vi "External Register Updated.vi"(4 "Register Value(s)":u16[](array[numeric]), 6 "String Value":string, 8 "error in (no error)":errorcluster, 9 "Value":dbl, 10 "Label":string, 11 "MB Slave in":refnum<class "Battery Pack.lvclass">) -> (0 "error out":errorcluster, 2 "Debug Cluster":cluster{string, string, "Value":dbl}, 3 "MB Slave out":refnum<class "Battery Pack.lvclass">)   [LabVIEW 2021, in "Battery Pack.lvclass"]
uses:
  Battery Pack.lvclass
  C:/Program Files (x86)/National Instruments/LabVIEW 2021/user.lib/S2 Labs/Module Framework/Modules/Base/Module.lvclass
  C:/Program Files (x86)/National Instruments/LabVIEW 2021/user.lib/S2 Labs/Module Framework/Modules/Modbus/Modbus Slave Base/Modbus Slave Base.lvclass
  <userlib>/S2 Labs/Queued State Machine/TypeDefs/Queue Message.ctl
  <userlib>/S2 Labs/Queued State Machine/TypeDefs/States.ctl
  <userlib>/S2 Labs/Module Framework/Modules/Base/Module.lvclass/Module.ctl
  <userlib>/S2 Labs/Queued State Machine/QSM.lvclass/QSM.ctl
  <userlib>/S2 Labs/Module Framework/Modules/Modbus/Modbus Slave Base/Modbus Slave Base.lvclass/Modbus Slave Base.ctl
  3c32b7f4-6e0b-45a0-8bc8-92411707fda7.vi
  a5158770-3295-4c9c-bae0-3194b8534535.vi
  f352f066-f63e-40b9-9452-5cd8e12a8467.vi
  5f4802e9-4a10-4382-9869-df42cea41124.vi
  <userlib>/S2 Labs/Module Framework/Modules/Base/Read Name.vi
  <userlib>/S2 Labs/Module Framework/Modules/Modbus/Modbus Slave Base/Read MB Ref.vi
  b984352d-4769-4dd1-9690-e9a5a354050f.vi
  0fd58ad7-8179-4fbb-beb2-807b76c45ab5.vi
  fadbf1c2-6df0-41ab-86c2-22b80328d9ad.vi
  a5158770-3295-4c9c-bae0-3194b8534535.vi/a5442550-30ab-4f7c-a4e8-4e040bcf3d57.vi
  <userlib>/S2 Labs/Module Framework/Modules/Base/Read Queue.vi
  a5158770-3295-4c9c-bae0-3194b8534535.vi/77abbf80-a0d7-431e-91bd-d2268efe8bf3.vi
  a5158770-3295-4c9c-bae0-3194b8534535.vi/7a27d807-84e4-485a-8ba6-289735576614.vi
  5f4802e9-4a10-4382-9869-df42cea41124.vi/a5442550-30ab-4f7c-a4e8-4e040bcf3d57.vi
  5f4802e9-4a10-4382-9869-df42cea41124.vi/77abbf80-a0d7-431e-91bd-d2268efe8bf3.vi
  5f4802e9-4a10-4382-9869-df42cea41124.vi/7a27d807-84e4-485a-8ba6-289735576614.vi
  0fd58ad7-8179-4fbb-beb2-807b76c45ab5.vi/a5442550-30ab-4f7c-a4e8-4e040bcf3d57.vi
  0fd58ad7-8179-4fbb-beb2-807b76c45ab5.vi/77abbf80-a0d7-431e-91bd-d2268efe8bf3.vi
  0fd58ad7-8179-4fbb-beb2-807b76c45ab5.vi/7a27d807-84e4-485a-8ba6-289735576614.vi
  fadbf1c2-6df0-41ab-86c2-22b80328d9ad.vi/a5442550-30ab-4f7c-a4e8-4e040bcf3d57.vi
  fadbf1c2-6df0-41ab-86c2-22b80328d9ad.vi/77abbf80-a0d7-431e-91bd-d2268efe8bf3.vi
  fadbf1c2-6df0-41ab-86c2-22b80328d9ad.vi/7a27d807-84e4-485a-8ba6-289735576614.vi
  <userlib>/S2 Labs/Queued State Machine/Enqueue Element.vi
  <userlib>/S2 Labs/Module Framework/Modules/Base/Get Module Queues Map.vi
  <userlib>/S2 Labs/Queued State Machine/Callback Notifier/Obtain Callback Notifier.vi
  <userlib>/S2 Labs/Queued State Machine/Callback Notifier/Release Reply Notifier.vi
  <vilib>/JDP Science/JSONtext/Variant to JSON Text.vi
  <userlib>/S2 Labs/Alarms and Events Toolkit/Alarms/Set User Event.vi
  <userlib>/S2 Labs/Queued State Machine/QSM.lvclass
  <userlib>/S2 Labs/Queued State Machine/Callback Notifier/Callback Notifier.lvclass
  <vilib>/JDP Science/JSONtext/LVClass Serializer/JSONtext LVClass Serializer.lvclass
  <userlib>/S2 Labs/Modbus Toolkit/Slave/S2L Modbus Slave.lvclass
  MB Slave Simulator Base/MB Slave Simulator Base.lvclass
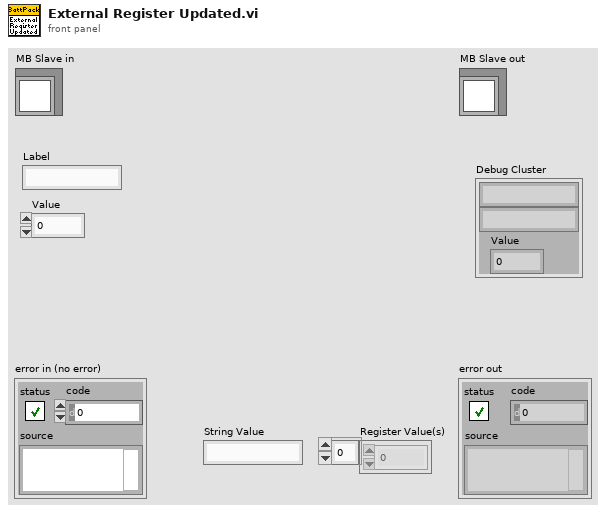
[diagram p1: front panel]
types:
  T1 = typedef "QSM.lvclass/Queue Message.ctl" = cluster{"State":T2, "Command":string, "Parameter":variant}
  T2 = typedef "QSM.lvclass/States.ctl" = enum16{"Waiting", "Init", "ExecCMD", "Read Config", "Write Config", "Launch", "Connect", "Recovery", "Clean Up", "Exit"}
  T3 = cluster{"Debug Message":string, string, "Value":dbl}
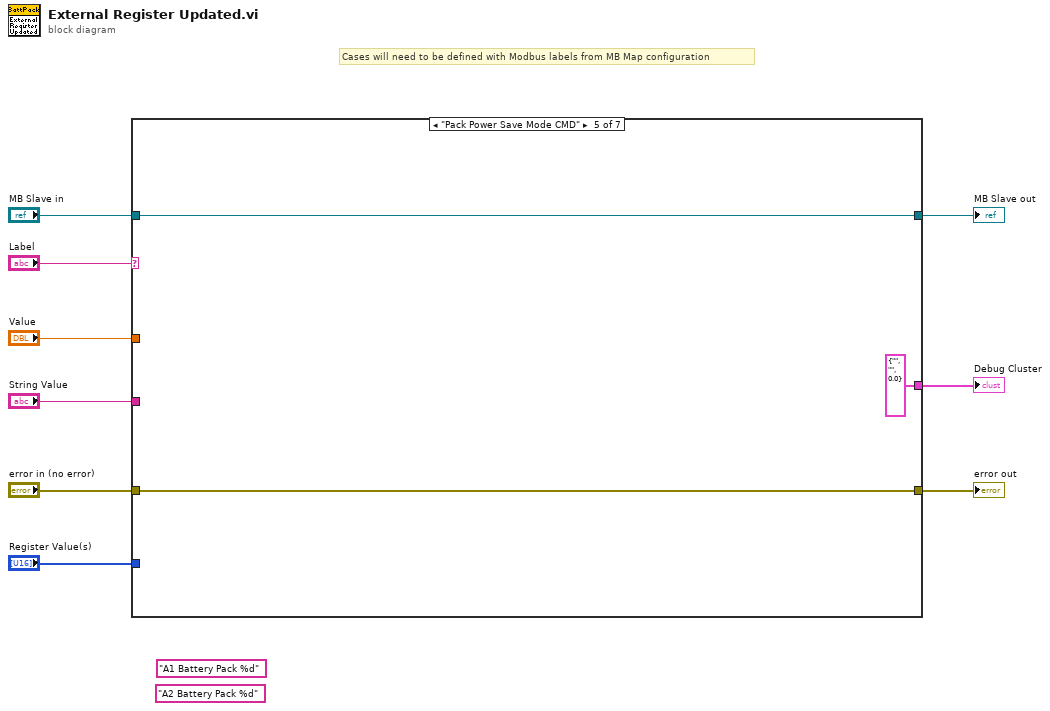
[diagram p0: block diagram]
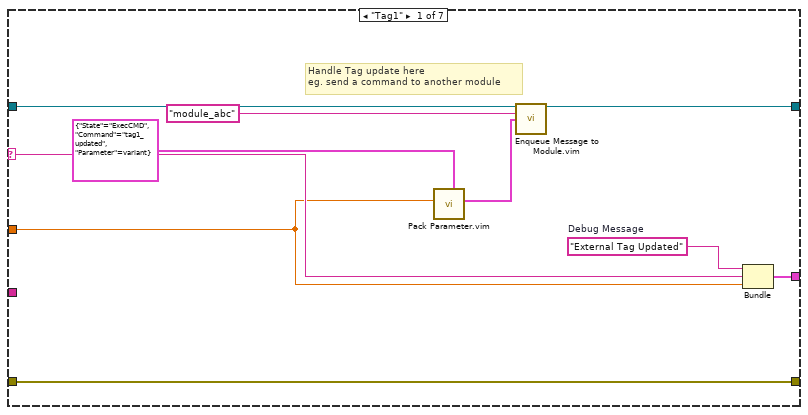
[diagram p2: hidden frame]
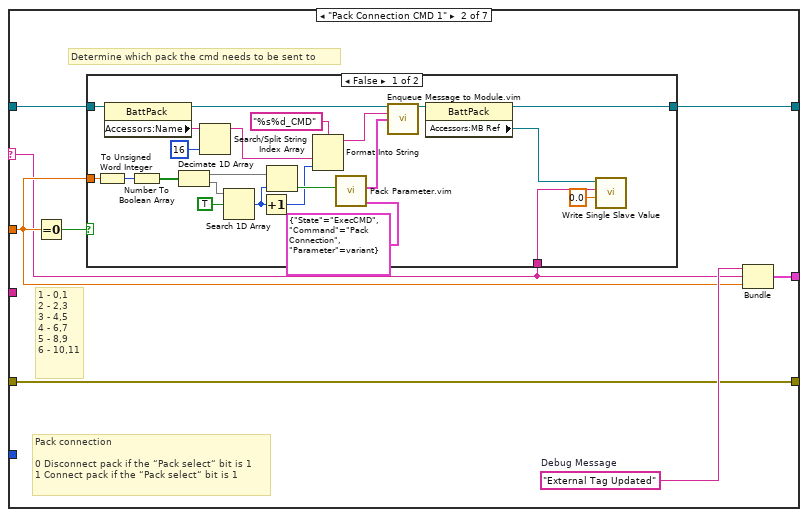
[diagram p3: hidden frame]
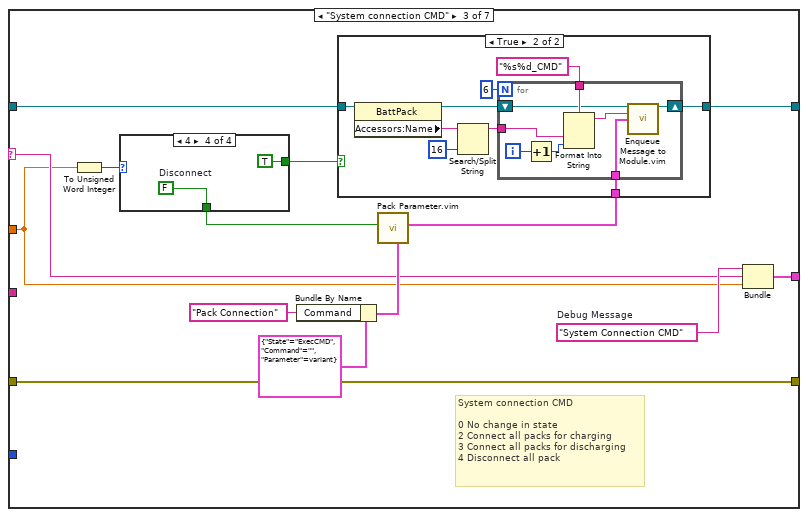
[diagram p5: hidden frame]
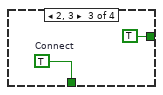
[diagram p8: hidden frame]
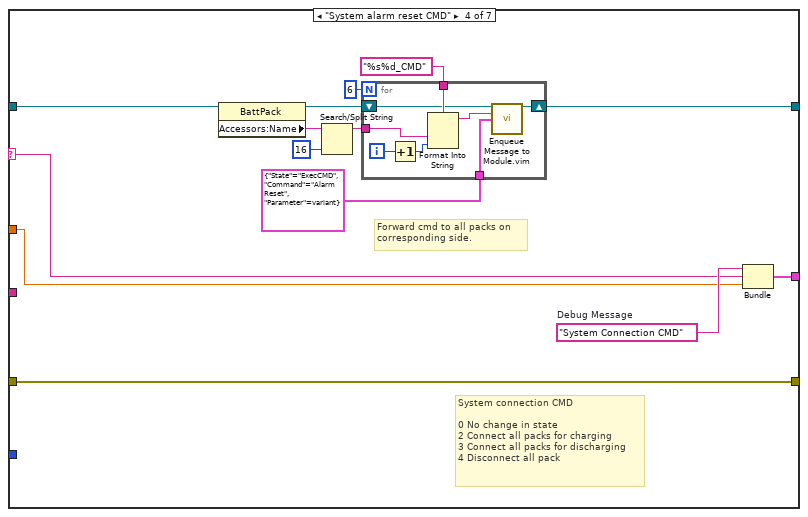
[diagram p10: hidden frame]
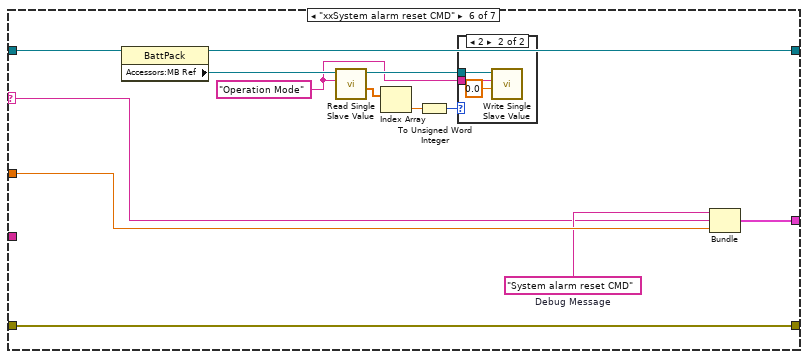
[diagram p11: hidden frame]
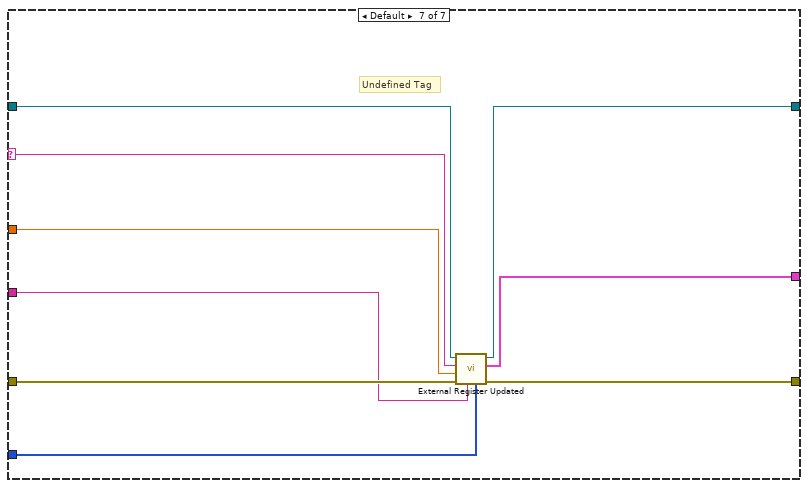
[diagram p13: hidden frame]
diagram:
  (unwired) "A2 Battery Pack %d"
  (unwired) "A1 Battery Pack %d"
  # "Cases will need to be defined with Modbus labels from MB Map configuration"
  n1 = case shown="\"Pack Power Save Mode CMD\"" "Label" {
    selector: "Label" -> [w18 w20 w57 w96 _ w121 w132]
    tunnel: [w16 w25 w63 w99 w110 w125 w137] -> w9
    tunnel: [w19 w27 w65 w101 T3 {"Debug Message"="", "", "Value"=0.0} ("Debug Cluster") w124 w136] -> w8
    tunnel: [w15 w24 w60 w97 w112 w120 w135] -> w7
    tunnel: "error in (no error)" -> [w16 w25 w63 w99 w110 w125 w134]
    tunnel: "Value" -> [w10 w22 w56 w95 _ w123 w133]
    tunnel: "MB Slave in" -> [w14 w23 w62 w98 w112 w119 w131]
    tunnel: "String Value" -> [_ _ _ _ _ _ w130]
    tunnel: "Register Value(s)" -> [_ _ _ _ _ _ w129]
    frame "Tag1" {
      w17 = "External Tag Updated"  # Debug Message
      # "Handle Tag update here\neg. send a command to another module"
      n2 = call "Pack Parameter.vim"("Message Cluster In"=T1 {"State"=enum."ExecCMD", "Command"="tag1_updated", "Parameter"=variant} ("Message"), "Parameter (string)"=w10) -> ("Message Cluster Out"=w11:T1)  [unwired: 9 in]
      n3 = call "Enqueue Message to Module.vim"("Module in"=w14, "Module Name (self)"="module_abc", "Message"=w11) -> ("Module out"=w15:refnum<class "Battery Pack.lvclass">)  [unwired: 7 in, 5 out]
      n4 = Bundle("Debug Message"=w17, w18, "Value"=w10) -> (w19:T3)  [unwired: 1 in]
    }
    frame "Pack Connection CMD 1" {
      w26 = "External Tag Updated"  # Debug Message
      # "1 - 0,1\n2 - 2,3\n3 - 4,5\n4 - 6,7\n5 - 8,9\n6 - 10,11"
      # "Pack connection\n\n0 Disconnect pack if the “Pack select“ bit is 1\n1 Connect pack if the “Pack select“ bit is 1"
      # "Determine which pack the cmd needs to be sent to"
      n5 = Equal To 0?(x=w22) -> (x = 0?=w21:bool)
      n6 = case shown="False" w21 {
        tunnel: [w31 w51] -> w24
        tunnel: w23 -> [w45 w51]
        tunnel: w22 -> [w44 _]
        tunnel: w20 -> [w29 _]
        frame False {
          n7 = To Unsigned Word Integer(number=w44) -> (unsigned 16bit integer=w43:u16)
          n8 = property class="BattPack"(reference=w45) -> (reference out=w46:refnum<class "Battery Pack.lvclass">, "Accessors:Name"=w48:string)  [unwired: 1 in, 1 out]
          n9 = Number To Boolean Array(number=w43) -> (Boolean array=w38:bool[])
          n10 = Decimate 1D Array(w38) -> (w41:bool[], w39:bool[])
          n11 = Search/Split String(string=w48, offset (0)=16) -> (substring before match=w35:string)  [unwired: 1 in, 2 out]
          n12 = Search 1D Array(1D array=w39, element=TRUE) -> (index of element=w42:i32)  [unwired: 1 in]
          n13 = Increment(x=w42) -> (x+1=w34:i32)
          n14 = Index Array(array=w41, index=w42) -> (element=w37:bool)
          n15 = Format Into String(format string="%s%d_CMD", w35, w34) -> (resulting string=w33:string)  [unwired: 2 in, 1 out]
          n16 = call "Pack Parameter.vim"("Message Cluster In"=T1 {"State"=enum."ExecCMD", "Command"="Pack Connection", "Parameter"=variant} ("Message"), "Parameter (string)"=w37) -> ("Message Cluster Out"=w49:T1)  [unwired: 9 in]
          n17 = call "Enqueue Message to Module.vim"("Module in"=w46, "Module Name (self)"=w33, "Message"=w49) -> ("Module out"=w32:refnum<class "Battery Pack.lvclass">)  [unwired: 7 in, 5 out]
          n18 = property class="BattPack"(reference=w32) -> (reference out=w31:refnum<class "Battery Pack.lvclass">, "Accessors:MB Ref"=w30:refnum<class "S2L Modbus Slave.lvclass">)  [unwired: 1 in, 1 out]
          n19 = call-dynamic "Write Single Slave Value.vi"("Value"=0.0, "Label"=w29, "S2L Modbus Slave in"=w30) -> ()  [unwired: 7 in, 2 out]
        }
        frame True {
          # "Deselect cmd, no action"
        }
      }
      n20 = Bundle("Debug Message"=w26, w20, "Value"=w22) -> (w27:T3)  [unwired: 1 in]
    }
    frame "System connection CMD" {
      w64 = "System Connection CMD"  # Debug Message
      # "System connection CMD\n\n0 No change in state\n2 Connect all packs for charging\n3 Connect all packs for discharging\n4 Disconnect all pack"
      n21 = To Unsigned Word Integer(number=w56) -> (unsigned 16bit integer=w55:u16)
      n22 = case shown="4" w55 {
        tunnel: [_ _ TRUE TRUE] -> w54
        tunnel: [_ _ w66 w68] -> w52
        frame Default {
        }
        frame 0, 1 {
        }
        frame 2, 3 {
          w66 = TRUE  # Connect
        }
        frame 4 {
          w68 = FALSE  # Disconnect
        }
      }
      n23 = Bundle By Name(cluster=T1 {"State"=enum."ExecCMD", "Command"="", "Parameter"=variant} ("Message"), "Command"="Pack Connection") -> (w58:T1)
      n24 = call "Pack Parameter.vim"("Message Cluster In"=w58, "Parameter (string)"=w52) -> ("Message Cluster Out"=w61:T1)  [unwired: 9 in]
      n25 = case shown="True" w54 {
        tunnel: w62 -> [w70 w79]
        tunnel: w61 -> [_ w72]
        tunnel: [w70 w71] -> w60
        frame False {
        }
        frame True {
          n26 = property class="BattPack"(reference=w79) -> (reference out=w73:refnum<class "Battery Pack.lvclass">, "Accessors:Name"=w74:string)  [unwired: 1 in, 1 out]
          n27 = Search/Split String(string=w74, offset (0)=16) -> (substring before match=w76:string)  [unwired: 1 in, 2 out]
          n28 = for {
            N: 6 -> [_]
            tunnel: w76 -> [w86]
            tunnel: "%s%d_CMD" ("format string") -> [w84]
            tunnel: w72 -> [w82]
            shift-right: [w81] -> w71
            shift-left: w73 -> [w83]
            i -> [w87]
            n29 = Increment(x=w87) -> (x+1=w85:i32)
            n30 = Format Into String(format string=w84, w86, w85) -> (resulting string=w80:string)  [unwired: 2 in, 1 out]
            n31 = call "Enqueue Message to Module.vim"("Module in"=w83, "Module Name (self)"=w80, "Message"=w82) -> ("Module out"=w81:refnum<class "Battery Pack.lvclass">)  [unwired: 7 in, 5 out]
          }
        }
      }
      n32 = Bundle("Debug Message"=w64, w57, "Value"=w56) -> (w65:T3)  [unwired: 1 in]
    }
    frame "System alarm reset CMD" {
      w100 = "System Connection CMD"  # Debug Message
      # "Forward cmd to all packs on\ncorresponding side."
      # "System connection CMD\n\n0 No change in state\n2 Connect all packs for charging\n3 Connect all packs for discharging\n4 Disconnect all pack"
      n33 = property class="BattPack"(reference=w98) -> (reference out=w89:refnum<class "Battery Pack.lvclass">, "Accessors:Name"=w90:string)  [unwired: 1 in, 1 out]
      n34 = Search/Split String(string=w90, offset (0)=16) -> (substring before match=w92:string)  [unwired: 1 in, 2 out]
      n35 = for {
        N: 6 -> [_]
        tunnel: w92 -> [w108]
        tunnel: "%s%d_CMD" ("format string") -> [w106]
        tunnel: T1 {"State"=enum."ExecCMD", "Command"="Alarm Reset", "Parameter"=variant} ("Message") -> [w104]
        shift-right: [w103] -> w97
        shift-left: w89 -> [w105]
        i -> [w109]
        n36 = Increment(x=w109) -> (x+1=w107:i32)
        n37 = Format Into String(format string=w106, w108, w107) -> (resulting string=w102:string)  [unwired: 2 in, 1 out]
        n38 = call "Enqueue Message to Module.vim"("Module in"=w105, "Module Name (self)"=w102, "Message"=w104) -> ("Module out"=w103:refnum<class "Battery Pack.lvclass">)  [unwired: 7 in, 5 out]
      }
      n39 = Bundle("Debug Message"=w100, w96, "Value"=w95) -> (w101:T3)  [unwired: 1 in]
    }
    frame "Pack Power Save Mode CMD" {
    }
    frame "xxSystem alarm reset CMD" {
      w116 = "Operation Mode"
      w122 = "System alarm reset CMD"  # Debug Message
      n40 = property class="BattPack"(reference=w119) -> (reference out=w120:refnum<class "Battery Pack.lvclass">, "Accessors:MB Ref"=w118:refnum<class "S2L Modbus Slave.lvclass">)  [unwired: 1 in, 1 out]
      n41 = call-dynamic "Read Single Slave Value.vi"("Label"=w116, "S2L Modbus Slave in"=w118) -> ("Value (s)"=w115:dbl[], "S2L Modbus Slave out"=w117:refnum<class "S2L Modbus Slave.lvclass">)  [unwired: 4 in, 4 out]
      n42 = Index Array(array=w115) -> (element=w114:dbl)  [unwired: 1 in]
      n43 = To Unsigned Word Integer(number=w114) -> (unsigned 16bit integer=w113:u16)
      n44 = case shown="2" w113 {
        tunnel: w117 -> [_ w128]
        tunnel: w116 -> [_ w127]
        frame Default {
        }
        frame 2 {
          n45 = call-dynamic "Write Single Slave Value.vi"("Value"=0.0, "Label"=w127, "S2L Modbus Slave in"=w128) -> ()  [unwired: 7 in, 2 out]
        }
      }
      n46 = Bundle("Debug Message"=w122, w121, "Value"=w123) -> (w124:T3)  [unwired: 1 in]
    }
    frame Default {
      # "Undefined Tag"
      n47 = call-parent "External Register Updated.vi"("Register Value(s)"=w129, "String Value"=w130, "error in (no error)"=w134, "Value"=w133, "Label"=w132, "MB Slave in"=w131) -> ("error out"=w137:errorcluster, "Debug Cluster"=w136:cluster{string, string, "Value":dbl}, "MB Slave out"=w135:refnum<class "Battery Pack.lvclass">)  [unwired: 3 in]
    }
  }
  "error out" <- w9
  "MB Slave out" <- w7
  "Debug Cluster" <- w8
